vi "Pike Loop.vi"() -> ()   [LabVIEW 2014]
uses:
  Pike Command.ctl
  Pike Mode.ctl
  Pike Indicators.ctl
  Pike State.ctl
  Common Code/Change Detect Int.vi
  Robot Global Data.vi
panel:
  in  "Pike Command":T1
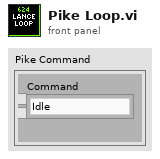
[diagram p1: front panel]
types:
  T1 = typedef "Pike Command.ctl" = cluster{"Command":T2}
  T2 = typedef "Pike Mode.ctl" = enum16{"Idle", "Auto Down", "Auto Up", "Manual Down", "Manual Up"}
  T3 = typedef "Pike Indicators.ctl" = cluster{"Motor Out":dbl, "Current":dbl, "Limit Switch":bool, "Current Limit":bool, "State":T4, "Command":T2}
  T4 = typedef "Pike State.ctl" = enum16{"Up", "Down", "Going Up", "Going Down"}
  T5 = typedef "WPI_DigitalInputDevRef.ctl" = cluster{"DevStatus":errorcluster, "DIO Channel":T6, "Controller":T7}
  T6 = typedef "FPGA_DIOChannel.ctl" = enum8{"DIO 0", "DIO 1", "DIO 2", "DIO 3", "DIO 4", "DIO 5", "DIO 6", "DIO 7", "DIO 8", "DIO 9", "DIO MXP 0", "DIO MXP 1", "DIO MXP 2", "DIO MXP 3", "DIO MXP 4", "DIO MXP 5", "DIO MXP 6", "DIO MXP 7", "DIO MXP 8", "DIO MXP 9", "DIO MXP 10", "DIO MXP 11", "DIO MXP 12", "DIO MXP 13", "DIO MXP 14", "DIO MXP 15", "Invalid"}
  T7 = typedef "FPGA_TypedefDigitalModule.ctl" = enum16{"Controller 1"}
  T8 = typedef "WPI_MotorControlDeviceRef.ctl" = cluster{"DeviceStatus":errorcluster, "Type":T9, "PWM":cluster{"Controller":T7, "PWM Channel":T10, "DeadBand":T11}, "CAN":cluster{"Device Number":u8, "Control Mode":T12, "Semaphore":T13, "Max Vout":dbl, "TalonSRX Control Mode":T14}, "Invert":bool, "TransformRef":T15, "InvTransformRef":T15}
  T9 = typedef "WPI_MotorControlType.ctl" = enum16{"PWM", "CAN", "CANTalonSRX"}
  T10 = typedef "FPGA_DIOPWMChannel.ctl" = enum8{"PWM 0", "PWM 1", "PWM 2", "PWM 3", "PWM 4", "PWM 5", "PWM 6", "PWM 7", "PWM 8", "PWM 9", "PWM MXP 0", "PWM MXP 1", "PWM MXP 2", "PWM MXP 3", "PWM MXP 4", "PWM MXP 5", "PWM MXP 6", "PWM MXP 7", "PWM MXP 8", "PWM MXP 9", "Invalid"}
  T11 = typedef "WPI_PWMDeadband.ctl" = cluster{"Name":string, "maxPositivePwm":i32, "minPositivePwm":i32, "centerPwm":i32, "maxNegativePwm":i32, "minNegativePwm":i32, "angularRange":u16}
  T12 = typedef "WPI_CANJaguar_ControlMode.ctl" = enum8{"Percent VBus", "Current", "Speed", "Position", "Voltage"}
  T13 = typedef "Semaphore RefNum" = refnum<k1>
  T14 = typedef "WPI_CANTalonSRX_APIControlMode.ctl" = enum8{"Percent VBus", "Speed", "Position", "Slave", "Unchanged / Invalid"}
  T15 = typedef "WPI_PWMTransform_ConPane.ctl" = refnum<vi>
  T16 = typedef "Dashboard Control Data.ctl" = cluster{"Cam Exposure":dbl, "Go to angle":dbl, "Steer PID Gains":cluster{"proportional gain (Kc)":dbl, "integral time (Ti, min)":dbl, "derivative time (Td, min)":dbl}, "Steer PID output Range":cluster{"output high":dbl, "output low":dbl}, "Pressure m \nValue":dbl, "Pressure b \nValue":dbl, "Roller Command Cluster ":T17, "Elevator":T18, "Encoder Control":T20, "Auton Settings":cluster{"Drive Dist Window Size":dbl}, "Drivetrain Settings":T21, "Pike":T22}
  T17 = typedef "Roller Control.ctl" = cluster{"Intake Speed":dbl, "Turn In Speed":dbl, "Unload Speed":dbl, "Turn Out Speed":dbl, "Ping Align Tolerance":dbl, "Tote Range Threshold":dbl, "Right Pot 0":dbl, "Pot Threshold":dbl, "Left Pot 0":dbl, "Manual 0s?":bool, "Right Pot Scale":dbl, "Left Pot Scale":dbl, "0 wait time":i32, "Zero Pots":bool, "Min Elevator Height":dbl, "Eject Time":dbl, "Eject US Threshold":dbl, "Anti-Twitch Time":u32, "Ping Caring Threshold":dbl, "Pot Diff Threshold":dbl, "Pinch Sustain":u32, "Absorb Give Up Threshold":dbl, "Untip In Threshold":dbl, "Untip Grab Range":dbl, "Ultrasonic Hold Time":u32, "Landscape Absorb Time":u32, "Pot Use Wait Time":u32, "Can Turn Stop Range":dbl, "Ignore Pressure":bool, "HP Load Speed":dbl}
  T18 = typedef "Elevator DB Control.ctl" = cluster{"PID Output Range":cluster{"output high":dbl, "output low":dbl}, "PID gains":cluster{"proportional gain (Kc)":dbl, "integral time (Ti, min)":dbl, "derivative time (Td, min)":dbl}, "Height Tolerance":sgl, " Encoder Constant":dbl, "Safe Mode Max Speed":sgl, "Eject Time":sgl, "Zeroing Speed":sgl, "Presets":T19, "Ping Detect Threshold":sgl, "Trashcan Detect Threshold":sgl, "Zero Filter Time":dbl, "Stabilizer Open Time":dbl, "Zero Creep Speed":dbl, "Max Current":dbl, "Current Trip Time":dbl, "Abort Pitch":dbl, "Finger m":dbl, "Finger b":dbl, "Finger max ":dbl, "Finger Stabilizer":dbl, "Finger Store":dbl, "Finger Stop Store":dbl, "Stabilizer Close Time":dbl, "HP Finger Store":dbl, "HP Finger Stop Store":dbl, "Finger min":dbl, "Unstick gain":dbl, "Roller Wait":dbl}
  T19 = typedef "Elevator Presets.ctl" = cluster{"Pickup 2 w/ Tote":sgl, "Pickup 2 w/ Trashcan":sgl, "Pickup 3 w/ Tote":sgl, "Pickup 3 w/ Trashcan":sgl, "Bottom":sgl, "Pickup 1 w/ Tote":sgl, "Pickup Trashcan":sgl, "Pickup 1 w/ Trashcan":sgl, "Eject":sgl, "Hold Low":sgl, "Step add height":sgl, "Untip Lift":dbl, "Drop Stack":dbl, "HP Load Hold":dbl, "HP Load Drop":dbl, "HP Load Finger":dbl, "HP Load Hold Can":dbl, "Store can max":dbl, "HP Drag Score":dbl, "HP Store can max":dbl, "HP Drag Finish":dbl, "HP Carry min":dbl, "HP Finger Anti-Crash":dbl, "Finger trashcan avoid":dbl}
  T20 = typedef "Encoder Control.ctl" = cluster{"Left Tick Constant":dbl, "Right Tick Constant":dbl, "Center Tick Constant":dbl, "Reset?":bool, "Y Dist":cluster{"PID gains":cluster{"proportional gain (Kc)":dbl, "integral time (Ti, min)":dbl, "derivative time (Td, min)":dbl}}, "X Dist":cluster{"PID gains":cluster{"proportional gain (Kc)":dbl, "integral time (Ti, min)":dbl, "derivative time (Td, min)":dbl}}, "Y Stop Thresh":dbl, "Y Stop Speed":dbl, "X Stop Thresh":dbl, "X Stop Speed":dbl}
  T21 = typedef "Drivetrain Settings.ctl" = cluster{"Gyro Tolerance":sgl, "Strafe Correct max steer":sgl, "Strafe Timer Wait":sgl, "Throttle Ramp (ms)":sgl, "Strafe Ramp (ms)":sgl, "Angular rate compensation":bool, "Throttle to Rate Scale":sgl, "Rate compensation gain":sgl, "Creep Steer":sgl, "Creep Throttle":sgl}
  T22 = typedef "Pike DB Controls.ctl" = cluster{"Down Speed":dbl, "Up Speed":dbl, "Max Down Time":dbl, "Max Up Time":dbl, "Current Limit":dbl}
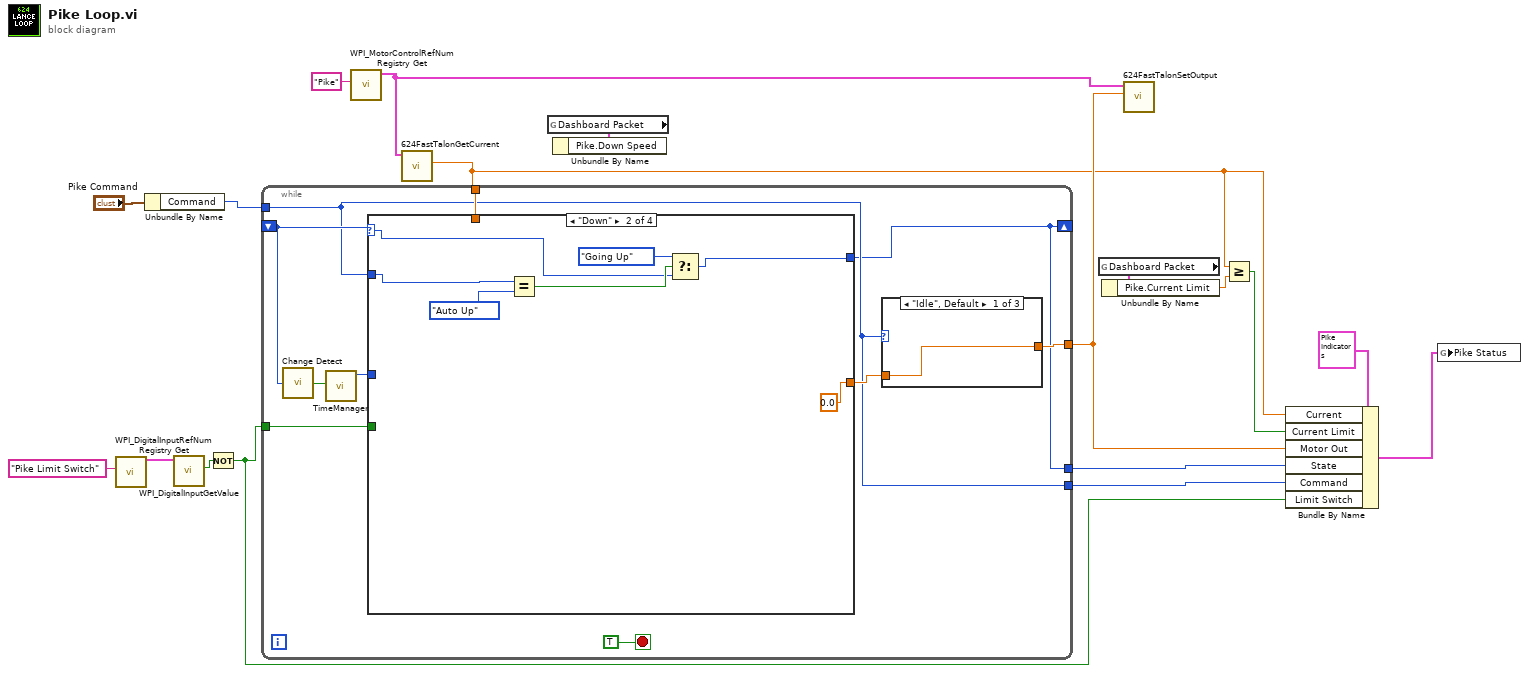
[diagram p0: block diagram]
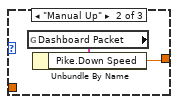
[diagram p2: hidden frame]
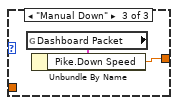
[diagram p3: hidden frame]
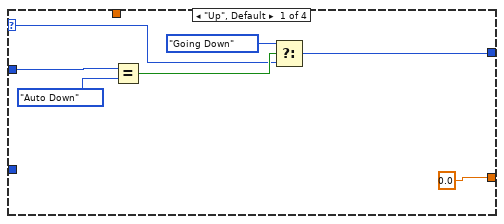
[diagram p4: hidden frame]
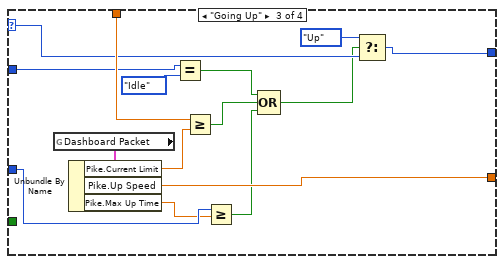
[diagram p5: hidden frame]
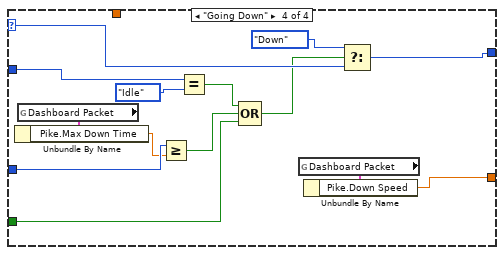
[diagram p6: hidden frame]
diagram:
  n1 = call <vilib>:"WPI_DigitalInputRefNum Registry Get.vi"("refnum name"="Pike Limit Switch") -> ("DigitalInputDevRef"=w12:T5)  [unwired: 9 in, 1 out]
  n2 = Unbundle By Name("Pike Command") -> ("Command"=w15:T2)
  n3 = call <vilib>:"WPI_DigitalInputGetValue.vi"("DigitalInputDevRef"=w12) -> ("Value"=w11:bool)  [unwired: 8 in, 2 out]
  n4 = Not(x=w11) -> (.not. x?=w7:bool)
  n5 = call <vilib>:"WPI_MotorControlRefNum Registry Get.vi"("refnum name"="Pike") -> ("MotorControlDevRef"=w14:T8)  [unwired: 9 in, 1 out]
  n6 = call "624FastTalonGetCurrent.vi"("CAN Talon SRX Ref"=w14) -> ("Current"=w2:dbl)  [unwired: 10 in]
  n7 = while {
    shift-right: [w19] -> _
    shift-left: _ -> [w23]
    tunnel: w15 -> [w20]
    tunnel: w2 -> [w27]
    tunnel: w7 -> [w26]
    tunnel: [w24] -> w8
    tunnel: [w20] -> w6
    tunnel: [w19] -> w5
    stop <- TRUE stop-if-true
    n8 = call-poly "Change Detect.vi"("In"=w23) -> ("Changed?"=w22:bool)
    n9 = call "TimeManager.vi"("Reset?"=w22) -> ("Time Since Reset"=w21:u32)  [unwired: 9 in, 1 out]
    n10 = case shown="\"Down\"" w23 {
      selector: w23 -> [w36 w42 w58 w74]
      tunnel: [0.0 0.0 w60 w75] -> w25
      tunnel: w20 -> [w39 w43 w53 w68]
      tunnel: [w34 w41 w56 w72] -> w19
      tunnel: w27 -> [_ _ w61 _]
      tunnel: w26 -> [_ _ _ w64]
      tunnel: w21 -> [_ _ w55 w70]
      frame "Up", Default {
        n11 = Equal?(x=w39, y=Pike_Mode."Auto Down") -> (x = y?=w37:bool)
        n12 = Select(t=Pike_State."Going Down", s=w37, f=w36) -> (s? t:f=w34:T4)
      }
      frame "Down" {
        n13 = Equal?(x=w43, y=Pike_Mode."Auto Up") -> (x = y?=w45:bool)
        n14 = Select(t=Pike_State."Going Up", s=w45, f=w42) -> (s? t:f=w41:T4)
      }
      frame "Going Up" {
        n15 = global read "Robot Global Data.vi" "Dashboard Packet"() -> (w62:T16)
        n16 = Unbundle By Name(w62) -> ("Pike.Current Limit"=w59:dbl, "Pike.Up Speed"=w60:dbl, "Pike.Max Up Time"=w54:dbl)
        n17 = Equal?(x=w53, y=Pike_Mode."Idle") -> (x = y?=w51:bool)
        n18 = Greater Or Equal?(x=w61, y=w59) -> (x >= y?=w50:bool)
        n19 = Greater Or Equal?(x=w55, y=w54) -> (x >= y?=w49:bool)
        n20 = Compound Arithmetic op=OR(w51, w50, w49) -> (w48:bool)
        n21 = Select(t=Pike_State."Up", s=w48, f=w58) -> (s? t:f=w56:T4)
      }
      frame "Going Down" {
        n22 = global read "Robot Global Data.vi" "Dashboard Packet"() -> (w71:T16)
        n23 = Unbundle By Name(w71) -> ("Pike.Max Down Time"=w69:dbl)
        n24 = Greater Or Equal?(x=w70, y=w69) -> (x >= y?=w65:bool)
        n25 = Equal?(x=w68, y=Pike_Mode."Idle") -> (x = y?=w66:bool)
        n26 = Compound Arithmetic op=OR(w66, w65, w64) -> (w63:bool)
        n27 = global read "Robot Global Data.vi" "Dashboard Packet"() -> (w76:T16)
        n28 = Unbundle By Name(w76) -> ("Pike.Down Speed"=w75:dbl)
        n29 = Select(t=Pike_State."Down", s=w63, f=w74) -> (s? t:f=w72:T4)
      }
    }
    n30 = case shown="\"Idle\", Default" w20 {
      tunnel: [w29 w30 w32] -> w24
      tunnel: w25 -> [w29 _ _]
      frame "Idle", Default {
      }
      frame "Manual Up" {
        n31 = global read "Robot Global Data.vi" "Dashboard Packet"() -> (w31:T16)
        n32 = Unbundle By Name(w31) -> ("Pike.Down Speed"=w30:dbl)
      }
      frame "Manual Down" {
        n33 = global read "Robot Global Data.vi" "Dashboard Packet"() -> (w33:T16)
        n34 = Unbundle By Name(w33) -> ("Pike.Down Speed"=w32:dbl)
      }
    }
  }
  n35 = global read "Robot Global Data.vi" "Dashboard Packet"() -> (w17:T16)
  n36 = Unbundle By Name(w17) -> ()  [unwired: 1 out]
  n37 = global read "Robot Global Data.vi" "Dashboard Packet"() -> (w4:T16)
  n38 = Unbundle By Name(w4) -> ("Pike.Current Limit"=w3:dbl)
  n39 = call "624FastTalonSetOutput.vi"("Output"=w8, "MotorControlDevRef"=w14) -> ()  [unwired: 8 in, 2 out]
  n40 = Greater Or Equal?(x=w2, y=w3) -> (x >= y?=w1:bool)
  n41 = Bundle By Name(cluster=T3 {"Motor Out"=0.0, "Current"=0.0, "Limit Switch"=FALSE, "Current Limit"=FALSE, "State"=enum."Going Up", "Command"=enum."Auto Up"} ("Pike Status"), "Current"=w2, "Current Limit"=w1, "Motor Out"=w8, "State"=w5, "Command"=w6, "Limit Switch"=w7) -> (w9:T3)
  n42 = global write "Robot Global Data.vi" "Pike Status"(w9) -> ()
